vi "gxml_XMLtoFlatString.vi"(8 "error in":errorcluster, 9 "Item XML Data":T2, 10 "Type Enum":T1, 11 "Item Type Desc":variant) -> (0 "error out":errorcluster, 2 "XML Data (Flat Str)":string)   [LabVIEW 2011, in "Third Party VIs.lvlib" / "GXML.lvlib"]
uses:
  GXML.lvlib
  <vilib>/Utility/VariantDataType/Type.ctl
  <vilib>/Utility/VariantDataType/VariantType.lvlib
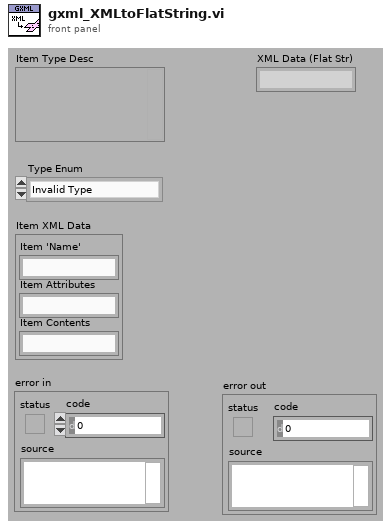
[diagram p1: front panel]
types:
  T1 = typedef "VariantType.lvlib/Type.ctl" = enum8{"Invalid Type", "Void", "I8", "I16", "I32", "I64", "U8", "U16", "U32", "U64", "Single Float", "Double Float", "Extended Float", "Single Complex", "Double Complex", "Extended Complex", "Enum U8", "Enum U16", "Enum U32", "Enum U64", "Single Float With Unit", "Double Float With Unit", "Extended Float With Unit", "Single Complex with Unit", "Double Complex with Unit", "Extended Complex with Unit", "Boolean", "String", "Path", "Picture", "Tag", "Array", "Cluster", "Variant", "LV Variant", "Waveform", "Timestamp", "Digital Waveform", "Digital Data", "ExpressData", "Refnum", "External Data", "VI", "Poly VI", "LabVIEW Class Instance", "Fixed Point"}
  T2 = cluster{"Item 'Name'":string, "Item Attributes":string, "Item Contents":string}
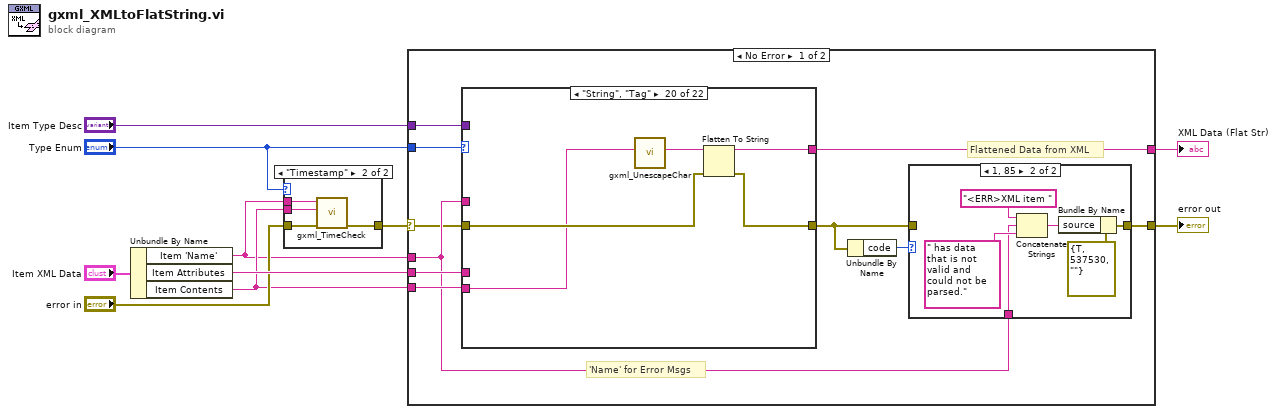
[diagram p0: block diagram]
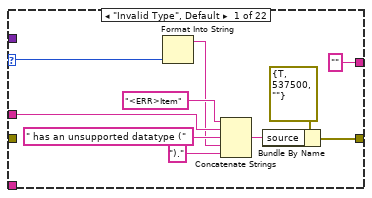
[diagram p3: hidden frame]
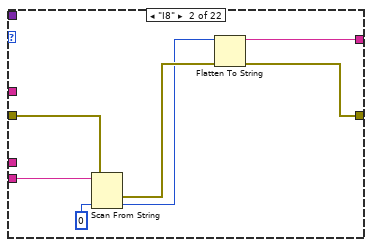
[diagram p4: hidden frame]
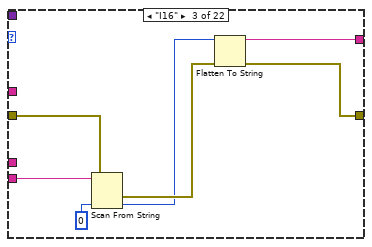
[diagram p5: hidden frame]
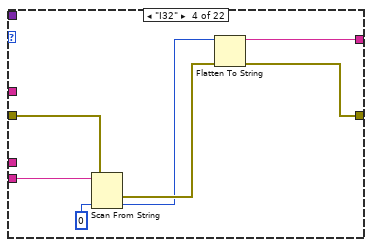
[diagram p6: hidden frame]
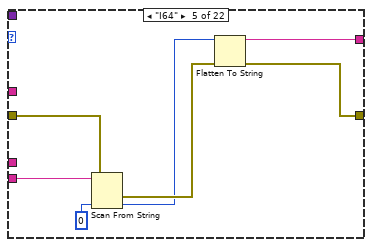
[diagram p7: hidden frame]
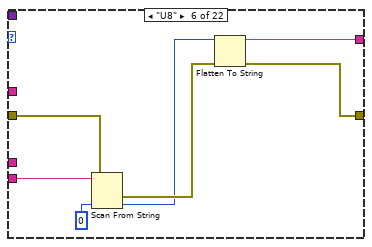
[diagram p8: hidden frame]
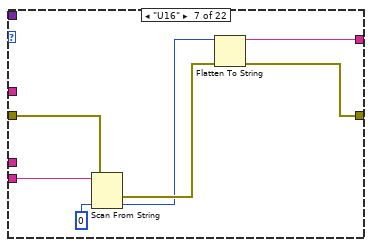
[diagram p9: hidden frame]
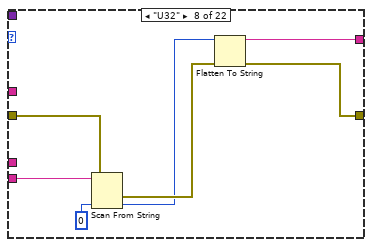
[diagram p10: hidden frame]
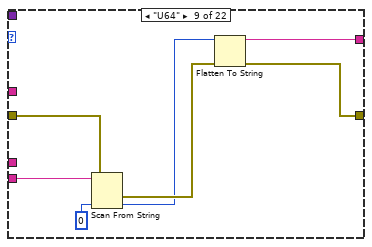
[diagram p11: hidden frame]
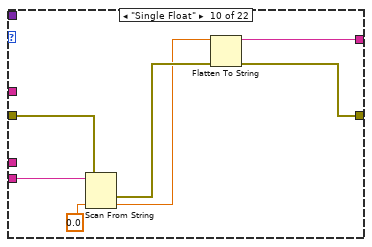
[diagram p12: hidden frame]
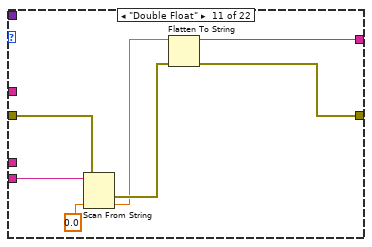
[diagram p13: hidden frame]
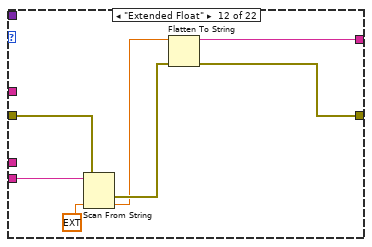
[diagram p14: hidden frame]
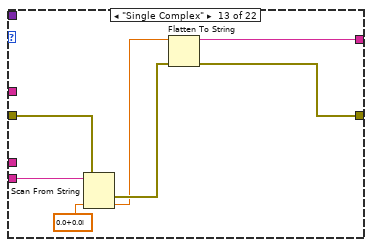
[diagram p15: hidden frame]
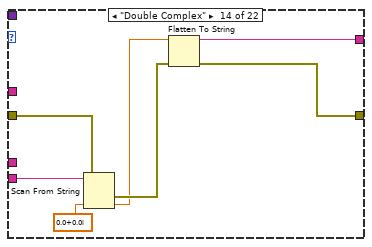
[diagram p16: hidden frame]
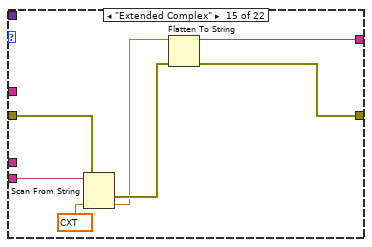
[diagram p17: hidden frame]
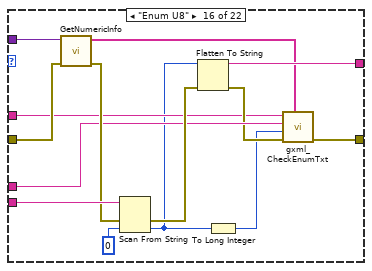
[diagram p18: hidden frame]
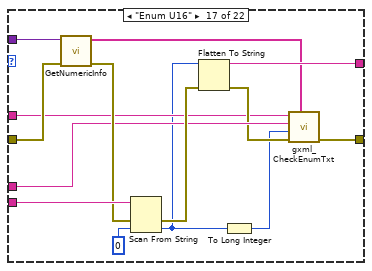
[diagram p19: hidden frame]
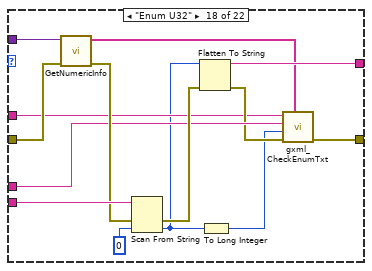
[diagram p20: hidden frame]
diagram:
  n1 = Unbundle By Name("Item XML Data") -> ("Item 'Name'"=w2:string, "Item Attributes"=w9:string, "Item Contents"=w3:string)
  n2 = case shown="\"Timestamp\"" "Type Enum" {
    tunnel: "error in" -> [w11 w15]
    tunnel: [w11 w14] -> w1
    tunnel: w3 -> [_ w13]
    tunnel: w2 -> [_ w12]
    frame "Invalid Type", Default {
    }
    frame "Timestamp" {
      n3 = call "gxml_TimeCheck.vi"("error in"=w15, "Time String"=w13, "Item Name"=w12) -> ("error out"=w14:errorcluster)  [unwired: 7 in]
    }
  }
  n4 = case shown="No Error" w1 {
    selector: w1 -> [w16 w210]
    tunnel: w9 -> [w25 _]
    tunnel: [w24 w210] -> w8
    tunnel: "Item Type Desc" -> [w23 _]
    tunnel: [w22 "" ("data string")] -> w6
    tunnel: "Type Enum" -> [w19 _]
    tunnel: w3 -> [w18 _]
    tunnel: w2 -> [w17 _]
    frame No Error {
      # "Flattened Data from XML"
      # "'Name' for Error Msgs"
      n5 = case shown="\"String\", \"Tag\"" w19 {
        selector: w19 -> [w38 _ _ _ _ _ _ _ _ _ _ _ _ _ _ _ _ _ _ _ _ _]
        tunnel: ["" ("data string") w46 w53 w60 w67 w74 w81 w88 w95 w104 w111 w118 w125 w132 w139 w145 w159 w173 w188 w193 w199 w207] -> w22
        tunnel: [w37 w45 w52 w59 w66 w73 w80 w87 w94 w105 w112 w119 w126 w133 w140 w146 w160 w174 w189 w194 w200 w208] -> w21
        tunnel: w18 -> [_ w48 w55 w62 w69 w76 w83 w90 w97 w102 w109 w116 w123 w130 w137 w154 w168 w182 w187 w190 w196 w206]
        tunnel: w16 -> [_ w47 w54 w61 w68 w75 w82 w89 w96 w99 w106 w113 w120 w127 w134 w150 w164 w178 w183 w192 w197 w202]
        tunnel: w25 -> [_ _ _ _ _ _ _ _ _ _ _ _ _ _ _ w148 w162 w176 _ _ _ _]
        tunnel: w23 -> [_ _ _ _ _ _ _ _ _ _ _ _ _ _ _ w151 w165 w179 _ _ _ _]
        tunnel: w17 -> [w36 _ _ _ _ _ _ _ _ _ _ _ _ _ _ w143 w157 w171 _ _ _ _]
        frame "Invalid Type", Default {
          n6 = Format Into String(w38) -> (resulting string=w35:string)  [unwired: 3 in, 1 out]
          n7 = Concatenate Strings("<ERR>Item" ("Format String"), w36, " has an unsupported datatype (" ("Format String"), w35, ")." ("string")) -> (w42:string)
          n8 = Bundle By Name(cluster=errorcluster {"status"=TRUE, "code"=537500, "source"=""} ("error in"), "source"=w42) -> (w37:errorcluster)
        }
        frame "I8" {
          n9 = Scan From String(input string=w48, error in=w47, default 1=i8 0) -> (error out=w44:errorcluster, output 1=w43:i8)  [unwired: 2 in, 2 out]
          n10 = Flatten To String(anything=w43, error in (no error)=w44) -> (data string=w46:string, error out=w45:errorcluster)  [unwired: 2 in, 1 out]
        }
        frame "I16" {
          n11 = Scan From String(input string=w55, error in=w54, default 1=i16 0) -> (error out=w51:errorcluster, output 1=w50:i16)  [unwired: 2 in, 2 out]
          n12 = Flatten To String(anything=w50, error in (no error)=w51) -> (data string=w53:string, error out=w52:errorcluster)  [unwired: 2 in, 1 out]
        }
        frame "I32" {
          n13 = Scan From String(input string=w62, error in=w61, default 1=0) -> (error out=w58:errorcluster, output 1=w57:i32)  [unwired: 2 in, 2 out]
          n14 = Flatten To String(anything=w57, error in (no error)=w58) -> (data string=w60:string, error out=w59:errorcluster)  [unwired: 2 in, 1 out]
        }
        frame "I64" {
          n15 = Scan From String(input string=w69, error in=w68, default 1=i64 0) -> (error out=w65:errorcluster, output 1=w64:i64)  [unwired: 2 in, 2 out]
          n16 = Flatten To String(anything=w64, error in (no error)=w65) -> (data string=w67:string, error out=w66:errorcluster)  [unwired: 2 in, 1 out]
        }
        frame "U8" {
          n17 = Scan From String(input string=w76, error in=w75, default 1=u8 0) -> (error out=w72:errorcluster, output 1=w71:u8)  [unwired: 2 in, 2 out]
          n18 = Flatten To String(anything=w71, error in (no error)=w72) -> (data string=w74:string, error out=w73:errorcluster)  [unwired: 2 in, 1 out]
        }
        frame "U16" {
          n19 = Scan From String(input string=w83, error in=w82, default 1=u16 0) -> (error out=w79:errorcluster, output 1=w78:u16)  [unwired: 2 in, 2 out]
          n20 = Flatten To String(anything=w78, error in (no error)=w79) -> (data string=w81:string, error out=w80:errorcluster)  [unwired: 2 in, 1 out]
        }
        frame "U32" {
          n21 = Scan From String(input string=w90, error in=w89, default 1=u32 0) -> (error out=w86:errorcluster, output 1=w85:u32)  [unwired: 2 in, 2 out]
          n22 = Flatten To String(anything=w85, error in (no error)=w86) -> (data string=w88:string, error out=w87:errorcluster)  [unwired: 2 in, 1 out]
        }
        frame "U64" {
          n23 = Scan From String(input string=w97, error in=w96, default 1=u64 0) -> (error out=w93:errorcluster, output 1=w92:u64)  [unwired: 2 in, 2 out]
          n24 = Flatten To String(anything=w92, error in (no error)=w93) -> (data string=w95:string, error out=w94:errorcluster)  [unwired: 2 in, 1 out]
        }
        frame "Single Float" {
          n25 = Scan From String(input string=w102, error in=w99, default 1=sgl 0.0) -> (error out=w101:errorcluster, output 1=w100:sgl)  [unwired: 2 in, 2 out]
          n26 = Flatten To String(anything=w100, error in (no error)=w101) -> (data string=w104:string, error out=w105:errorcluster)  [unwired: 2 in, 1 out]
        }
        frame "Double Float" {
          n27 = Scan From String(input string=w109, error in=w106, default 1=0.0) -> (error out=w108:errorcluster, output 1=w107:dbl)  [unwired: 2 in, 2 out]
          n28 = Flatten To String(anything=w107, error in (no error)=w108) -> (data string=w111:string, error out=w112:errorcluster)  [unwired: 2 in, 1 out]
        }
        frame "Extended Float" {
          n29 = Scan From String(input string=w116, error in=w113, default 1=ext 0.0) -> (error out=w115:errorcluster, output 1=w114:ext)  [unwired: 2 in, 2 out]
          n30 = Flatten To String(anything=w114, error in (no error)=w115) -> (data string=w118:string, error out=w119:errorcluster)  [unwired: 2 in, 1 out]
        }
        frame "Single Complex" {
          n31 = Scan From String(input string=w123, error in=w120, default 1=csg 0.0+0.0i) -> (error out=w122:errorcluster, output 1=w121:csg)  [unwired: 2 in, 2 out]
          n32 = Flatten To String(anything=w121, error in (no error)=w122) -> (data string=w125:string, error out=w126:errorcluster)  [unwired: 2 in, 1 out]
        }
        frame "Double Complex" {
          n33 = Scan From String(input string=w130, error in=w127, default 1=cdb 0.0+0.0i) -> (error out=w129:errorcluster, output 1=w128:cdb)  [unwired: 2 in, 2 out]
          n34 = Flatten To String(anything=w128, error in (no error)=w129) -> (data string=w132:string, error out=w133:errorcluster)  [unwired: 2 in, 1 out]
        }
        frame "Extended Complex" {
          n35 = Scan From String(input string=w137, error in=w134, default 1=cxt 0.0+0.0i) -> (error out=w136:errorcluster, output 1=w135:cxt)  [unwired: 2 in, 2 out]
          n36 = Flatten To String(anything=w135, error in (no error)=w136) -> (data string=w139:string, error out=w140:errorcluster)  [unwired: 2 in, 1 out]
        }
        frame "Enum U8" {
          n37 = call <vilib>:"GetNumericInfo.vi"("error in (no error)"=w150, "Variant"=w151) -> ("error out"=w149:errorcluster, "EnumNames"=w144:string[])  [unwired: 6 in, 2 out]
          n38 = Scan From String(input string=w154, error in=w149, default 1=u8 0) -> (error out=w152:errorcluster, output 1=w142:u8)  [unwired: 2 in, 2 out]
          n39 = Flatten To String(anything=w142, error in (no error)=w152) -> (data string=w145:string, error out=w147:errorcluster)  [unwired: 2 in, 1 out]
          n40 = To Long Integer(number=w142) -> (32bit integer=w141:i32)
          n41 = call "gxml_CheckEnumTxt.vi"("EnumNames"=w144, "error in"=w147, "EnumVal"=w141, "Item Attributes"=w148, "Item Name"=w143) -> ("error out"=w146:errorcluster)  [unwired: 6 in]
        }
        frame "Enum U16" {
          n42 = call <vilib>:"GetNumericInfo.vi"("error in (no error)"=w164, "Variant"=w165) -> ("error out"=w163:errorcluster, "EnumNames"=w158:string[])  [unwired: 6 in, 2 out]
          n43 = Scan From String(input string=w168, error in=w163, default 1=u16 0) -> (error out=w166:errorcluster, output 1=w155:u16)  [unwired: 2 in, 2 out]
          n44 = Flatten To String(anything=w155, error in (no error)=w166) -> (data string=w159:string, error out=w161:errorcluster)  [unwired: 2 in, 1 out]
          n45 = To Long Integer(number=w155) -> (32bit integer=w156:i32)
          n46 = call "gxml_CheckEnumTxt.vi"("EnumNames"=w158, "error in"=w161, "EnumVal"=w156, "Item Attributes"=w162, "Item Name"=w157) -> ("error out"=w160:errorcluster)  [unwired: 6 in]
        }
        frame "Enum U32" {
          n47 = call <vilib>:"GetNumericInfo.vi"("error in (no error)"=w178, "Variant"=w179) -> ("error out"=w177:errorcluster, "EnumNames"=w172:string[])  [unwired: 6 in, 2 out]
          n48 = Scan From String(input string=w182, error in=w177, default 1=u32 0) -> (error out=w180:errorcluster, output 1=w170:u32)  [unwired: 2 in, 2 out]
          n49 = Flatten To String(anything=w170, error in (no error)=w180) -> (data string=w173:string, error out=w175:errorcluster)  [unwired: 2 in, 1 out]
          n50 = To Long Integer(number=w170) -> (32bit integer=w169:i32)
          n51 = call "gxml_CheckEnumTxt.vi"("EnumNames"=w172, "error in"=w175, "EnumVal"=w169, "Item Attributes"=w176, "Item Name"=w171) -> ("error out"=w174:errorcluster)  [unwired: 6 in]
        }
        frame "Boolean" {
          n52 = Scan From String(input string=w187, error in=w183, default 1=FALSE) -> (error out=w185:errorcluster, output 1=w184:bool)  [unwired: 2 in, 2 out]
          n53 = Flatten To String(anything=w184, error in (no error)=w185) -> (data string=w188:string, error out=w189:errorcluster)  [unwired: 2 in, 1 out]
        }
        frame "String", "Tag" {
          n54 = call "gxml_UnescapeChar.vi"("XML In"=w190) -> ("XML Out"=w191:string)  [unwired: 10 in]
          n55 = Flatten To String(anything=w191, error in (no error)=w192) -> (data string=w193:string, error out=w194:errorcluster)  [unwired: 2 in, 1 out]
        }
        frame "Path" {
          n56 = call "gxml_UnescapeChar.vi"("XML In"=w196) -> ("XML Out"=w195:string)  [unwired: 10 in]
          n57 = String To Path(string=w195) -> (path=w198:path)
          n58 = Flatten To String(anything=w198, error in (no error)=w197) -> (data string=w199:string, error out=w200:errorcluster)  [unwired: 2 in, 1 out]
        }
        frame "Timestamp" {
          n59 = Scan From String(format string="%<%H:%M:%S %x>T", input string=w206, error in=w202, default 1=timestamp(0 s since 1904-01-01) ("time stamp")) -> (error out=w203:errorcluster, output 1=w205:timestamp)  [unwired: 1 in, 2 out]
          n60 = Flatten To String(anything=w205, error in (no error)=w203) -> (data string=w207:string, error out=w208:errorcluster)  [unwired: 2 in, 1 out]
        }
      }
      n61 = Unbundle By Name(w21) -> ("code"=w20:i32)
      n62 = case shown="1, 85" w20 {
        tunnel: w21 -> [w26 _]
        tunnel: [w26 w29] -> w24
        tunnel: w17 -> [_ w27]
        frame Default {
        }
        frame 1, 85 {
          n63 = Concatenate Strings("<ERR>XML item " ("Format String"), w27, " has data that is not valid and could not be parsed." ("Format String")) -> (w30:string)
          n64 = Bundle By Name(cluster=errorcluster {"status"=TRUE, "code"=537530, "source"=""} ("error in"), "source"=w30) -> (w29:errorcluster)
        }
      }
    }
    frame Error {
    }
  }
  "error out" <- w8
  "XML Data (Flat Str)" <- w6
